vi "AddTitleToPNG.vi"(8 "error in (no error)":errorcluster, 10 "Title String":string, 11 "PNG File":path) -> (0 "error out":errorcluster)   [LabVIEW 2020, in "VIDiffScreenshots.lvlib"]
uses:
  VIDiffScreenshots.lvlib
  ImageMagic/Label Position.ctl
  ImageMagic/VIDiffImageMagic.lvlib
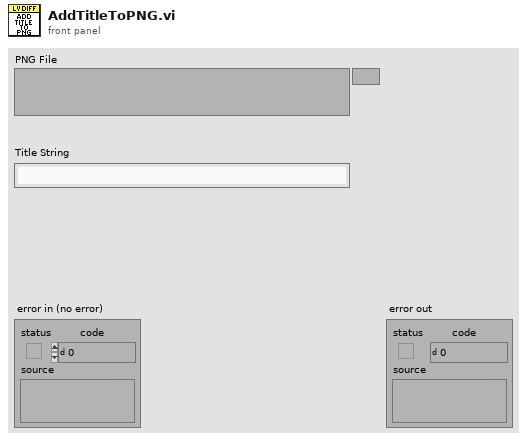
[diagram p1: front panel]
types:
  T1 = typedef "VIDiffImageMagic.lvlib/Label Position.ctl" = enum16{"Above", "Below"}
  T2 = cluster{"Font Name":string, "Size":i16, "Strikeout?":bool, "Italic?":bool, "Underline?":bool, "Bold?":bool}
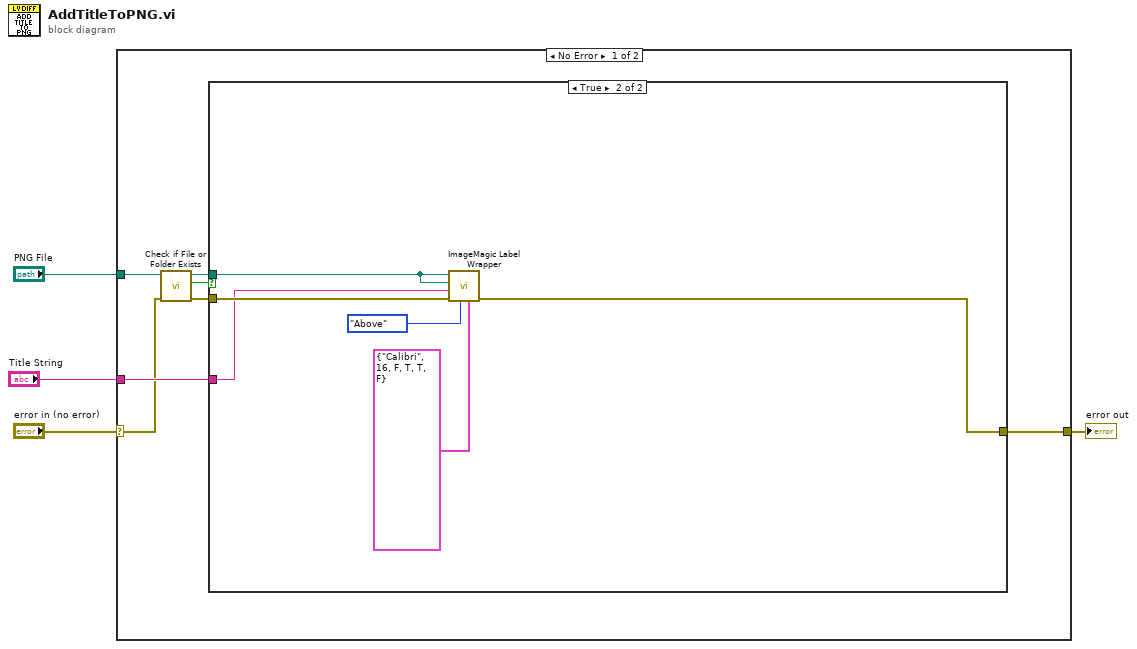
[diagram p0: block diagram]
diagram:
  n1 = case shown="No Error" "error in (no error)" {
    selector: "error in (no error)" -> [w6 w19]
    tunnel: "PNG File" -> [w9 _]
    tunnel: [w10 w19] -> w2
    tunnel: "Title String" -> [w11 _]
    frame No Error {
      n2 = call <vilib>:"Check if File or Folder Exists.vi"("error in (no error)"=w6, "path"=w9) -> ("error out"=w7:errorcluster, "file or folder exists?"=w5:bool, "dup path"=w8:path)  [unwired: 7 in]
      n3 = case shown="True" w5 {
        tunnel: w11 -> [_ w15]
        tunnel: [w12 w17] -> w10
        tunnel: w8 -> [_ w16]
        tunnel: w7 -> [w12 w18]
        frame False {
        }
        frame True {
          n4 = call "ImageMagic Label Wrapper.vi"("Font"=T2 {"Font Name"="Calibri", "Size"=16, "Strikeout?"=FALSE, "Italic?"=TRUE, "Underline?"=TRUE, "Bold?"=FALSE}, "Label Position"=Label_Position."Above", "error in (no error)"=w18, "Text"=w15, "Output File"=w16, "Input File"=w16) -> ("error out"=w17:errorcluster)  [unwired: 5 in]
        }
      }
    }
    frame Error {
    }
  }
  "error out" <- w2
